vi "Interpolate RGB Color.vi"(8 "Proportion":dbl(slide) scale=0.0..1.0, 10 "Target Color":u32(colorbox)=9502720, 11 "Base Color":u32(colorbox)=2829099) -> (3 "Result Color":u32(colorbox)=2829099)   [LabVIEW 2015]
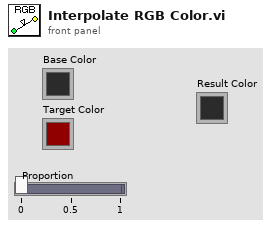
[diagram p1: front panel]
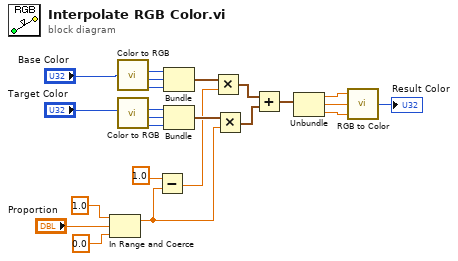
[diagram p0: block diagram]
diagram:
  n1 = In Range and Coerce(upper limit=1.0, x="Proportion", lower limit=0.0) -> (coerced(x)=w1:dbl)  [unwired: 1 out]
  n2 = call <vilib>:"Color to RGB.vi"("Color"="Base Color") -> ("R"=w20:u8, "G"=w19:u8, "B"=w18:u8)  [unwired: 1 out]
  n3 = call <vilib>:"Color to RGB.vi"("Color"="Target Color") -> ("R"=w15:u8, "G"=w16:u8, "B"=w17:u8)  [unwired: 1 out]
  n4 = Subtract(x=1.0, y=w1) -> (x-y=w2:dbl)
  n5 = Bundle("R"=w20, "G"=w19, "B"=w18) -> (w14:cluster{"R":u8, "G":u8, "B":u8})  [unwired: 1 in]
  n6 = Bundle("R"=w15, "G"=w16, "B"=w17) -> (w13:cluster{"R":u8, "G":u8, "B":u8})  [unwired: 1 in]
  n7 = Multiply(x=w14, y=w2) -> (x*y=w12:cluster{"R":dbl, "G":dbl, "B":dbl})
  n8 = Multiply(x=w13, y=w1) -> (x*y=w11:cluster{"R":dbl, "G":dbl, "B":dbl})
  n9 = Add(x=w12, y=w11) -> (x+y=w7:cluster{"R":dbl, "G":dbl, "B":dbl})
  n10 = Unbundle(w7) -> ("R"=w6:dbl, "G"=w5:dbl, "B"=w4:dbl)
  n11 = call <vilib>:"RGB to Color.vi"("B"=w4, "G"=w5, "R"=w6) -> ("Color"=→"Result Color":u32)
